vi "Set XY Graph X Mapping.vi"(8 "error in (no error)":errorcluster, 10 "X Scale Mapping":T1 items=["Linear", "Logarithmic"], 11 "graph_utilities in":refnum<class "graph_utilities.lvclass">) -> (0 "error out":errorcluster, 3 "graph_utilities out":refnum<class "graph_utilities.lvclass">)   [LabVIEW 2019, in "graph_utilities.lvclass"]
doc: "Set the X Scale Mapping (linear or logarithmic)."
uses:
  graph_utilities.lvclass
  Typedefs/Scale Mapping --enum.ctl
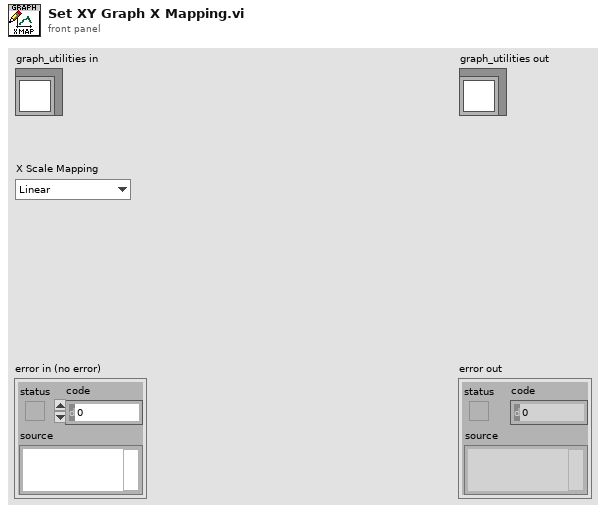
[diagram p1: front panel]
types:
  T1 = typedef "graph_utilities.lvclass/Scale Mapping --enum.ctl" = u16
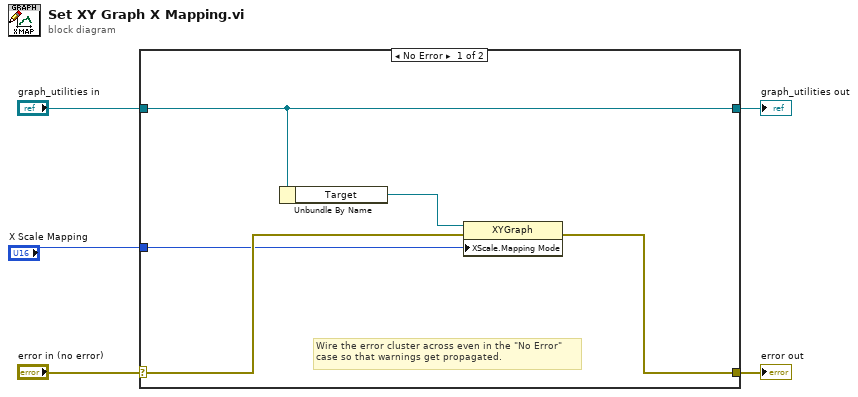
[diagram p0: block diagram]
diagram:
  n1 = case shown="No Error" "error in (no error)" {
    selector: "error in (no error)" -> [w8 w12]
    tunnel: [w7 w12] -> w4
    tunnel: [w10 w11] -> w2
    tunnel: "graph_utilities in" -> [w10 w11]
    tunnel: "X Scale Mapping" -> [w6 _]
    frame No Error {
      # "Wire the error cluster across even in the \"No Error\"\ncase so that warnings get propagated."
      n2 = Unbundle By Name(w10) -> ("Target"=w9:refnum<vi>)
      n3 = property on="Property Node" class="XYGraph"(reference=w9, error in=w8, "XScale.Mapping Mode"=w6) -> (error out=w7:errorcluster)  [unwired: 1 out]
    }
    frame Error {
    }
  }
  "error out" <- w4
  "graph_utilities out" <- w2
